vi "Chart GUI.vi"() -> ()   [LabVIEW 2020, in "VolatusGUI.lvlib" / "Historian Charting Manager.lvclass"]
uses:
  Historian Charting Manager.lvclass
  Historian Charting Manager.lvclass/Historian Charting Manager.ctl
panel:
  in  "HistorianChart":T1={"Config"=FALSE, "Time"="5 min", "Lock Time"=TRUE, "Plots"=[{"Channel"="", "Value"=0.0, "Color"=16777215, "Scale"=FALSE, "Visible"=FALSE}, {"Channel"="", "Value"=0.0, "Color"=16719378, "Scale"=FALSE, "Visible"=FALSE}, {"Channel"="", "Value"=0.0, "Color"=16756736, "Scale"=FALSE, "Visible"=FALSE}, {"Channel"="", "Value"=0.0, "Color"=16772394, "Scale"=FALSE, "Visible"=FALSE}, {"Channel"="", "Value"=0.0, "Color"=3538688, "Scale"=FALSE, "Visible"=FALSE}, {"Channel"="", "Value"=0.0, "Color"=65511, "Scale"=FALSE, "Visible"=FALSE}, {"Channel"="", "Value"=0.0, "Color"=4347135, "Scale"=FALSE, "Visible"=FALSE}, {"Channel"="", "Value"=0.0, "Color"=11534575, "Scale"=FALSE, "Visible"=FALSE}, {"Channel"="", "Value"=0.0, "Color"=10122868, "Scale"=FALSE, "Visible"=FALSE}, {"Channel"="", "Value"=0.0, "Color"=9078116, "Scale"=FALSE, "Visible"=FALSE}, {"Channel"="", "Value"=0.0, "Color"=8166004, "Scale"=FALSE, "Visible"=FALSE}, {"Channel"="", "Value"=0.0, "Color"=7115402, "Scale"=FALSE, "Visible"=FALSE}, {"Channel"="", "Value"=0.0, "Color"=6583690, "Scale"=FALSE, "Visible"=FALSE}, {"Channel"="", "Value"=0.0, "Color"=8938634, "Scale"=FALSE, "Visible"=FALSE}, {"Channel"="", "Value"=0.0, "Color"=8684676, "Scale"=FALSE, "Visible"=FALSE}], "Graph"=[], "Selection"=""} {"Plots"."Value" format="%.1f"}
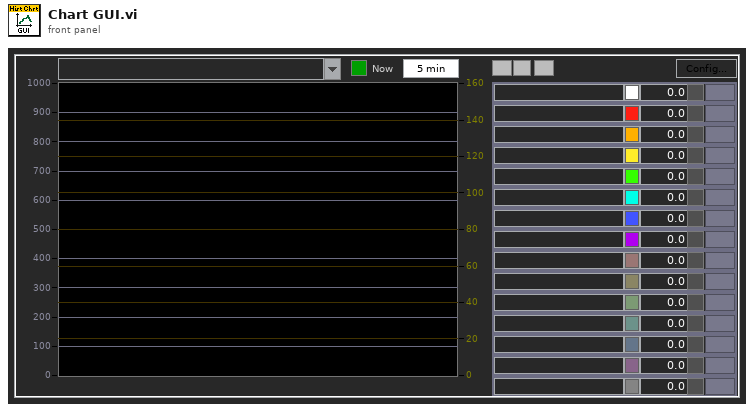
[diagram p1: front panel]
types:
  T1 = cluster{"Config":bool, "Time":string, "Lock Time":bool, "Plots":cluster{"Channel":string, "Value":dbl, "Color":u32, "Scale":bool, "Visible":bool}[], "Graph":cluster{dbl[], dbl[]}[], "Selection":string}
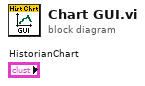
[diagram p0: block diagram]
diagram:
